vi "to string.vi"(8 "error in":errorcluster, 11 "fixed channel configuration in":refnum<class "fixed channel configuration.lvclass">) -> (0 "error out":errorcluster, 1 "data":string, 2 "version":string, 3 "fixed channel configuration out":refnum<class "fixed channel configuration.lvclass">)   [LabVIEW 2013, in "fixed channel configuration.lvclass"]
doc: "Provides an interface for saving a module configuration to a file or other serialized data source. It is recommended that all children of this class store data in two sets--data required for its own initialization, and any data required for parent initialization--and that each implementation uses the <b>Call Parent Method</b> primitive to serialize parent information.\nNI Tag Bus Module Framework 1.0.3.43\nNI Systems Engineering"
uses:
  fixed channel configuration.lvclass
  <vilib>/NI/DCAF/Tag Editor Core/control module/configuration/control module configuration.lvclass
  <vilib>/NI/Configuration Framework/serializable configuration/NISE_CEF_serializable configuration.lvclass
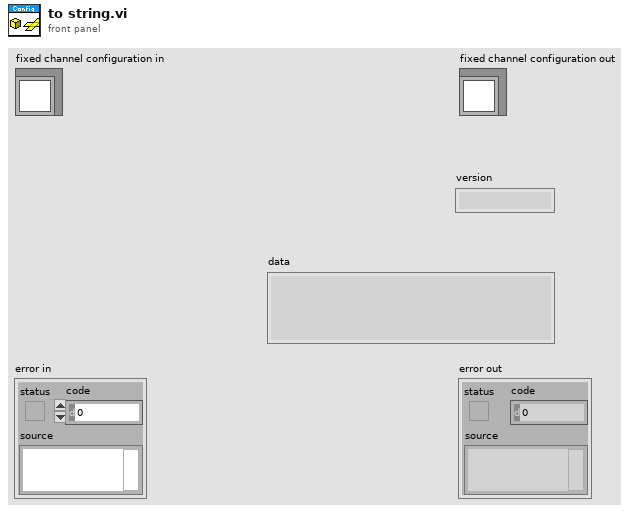
[diagram p1: front panel]
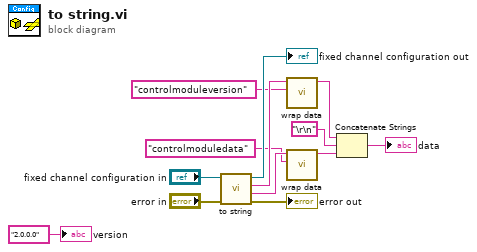
[diagram p0: block diagram]
diagram:
  n1 = call-parent "to string.vi"("error in"="error in", "fixed channel configuration in"="fixed channel configuration in") -> ("error out"=→"error out":errorcluster, "data"=w5:string, "version"=w4:string, "fixed channel configuration out"=→"fixed channel configuration out":refnum<class "fixed channel configuration.lvclass">)  [unwired: 6 in]
  n2 = call <vilib>:"wrap data.vi"("identifier"="controlmoduleversion", "data to wrap"=w4) -> ("wrapped data"=w6:string)  [unwired: 9 in]
  n3 = call <vilib>:"wrap data.vi"("identifier"="controlmoduledata", "data to wrap"=w5) -> ("wrapped data"=w7:string)  [unwired: 9 in]
  n4 = Concatenate Strings(w6, "\r\n", w7) -> (→"data":string)
  "version" <- "2.0.0.0" ("version")
